vi "Compound_Arithmatic.vi"() -> ()   [LabVIEW 2020]
panel:
  in  "D":dbl
  in  "C":dbl
  in  "B":dbl
  in  "A":dbl
  out "Multiplication":dbl
  out "Addition":dbl
  # "Add and Multiply more than two numeric inputs, i.e., Compound Arithmatic"
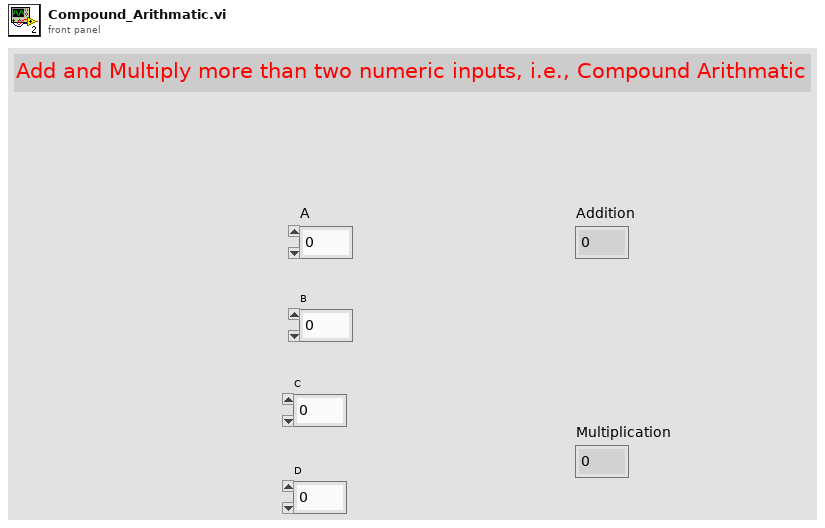
[diagram p1: front panel]
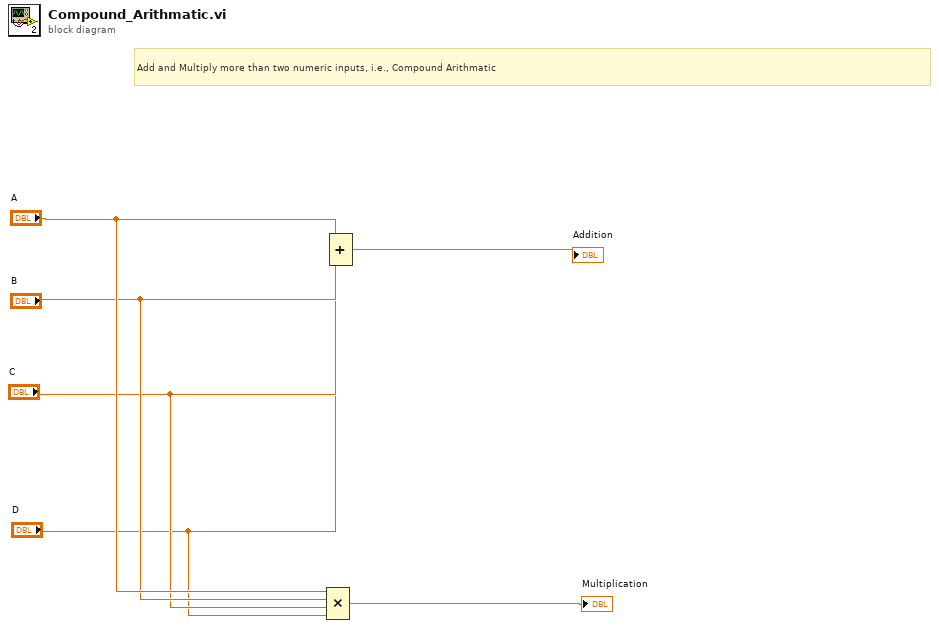
[diagram p0: block diagram]
diagram:
  # "Add and Multiply more than two numeric inputs, i.e., Compound Arithmatic"
  n1 = Compound Arithmetic op=MULTIPLY("A", "B", "C", "D") -> (→"Multiplication":dbl)
  n2 = Compound Arithmetic op=ADD("A", "B", "C", "D") -> (→"Addition":dbl)
